vi "Tabelle in die einzelnen Seiten zerlegen.vi"(5 "alternative Datei":string, 6 "Aktion":T1, 7 "Translate.exe":bool, 8 "error in (no error)":errorcluster caption="Fehler (Eingang, kein Fehler)", 9 "Sprachseite":string[][](array[string]), 10 "Eingang":string[][](array[string]), 11 "Index (Seite)":i32) -> (0 "error out":errorcluster caption="Fehler (Ausgang)", 2 "all rows":string[][][](array[string]), 3 "Sprachliste":string[][](array[string]))   [LabVIEW 2020, in "Sprachverwaltung.lvlib"]
doc: "Mit diesen VI kann man die Sprachdatei in den Einzelnen Seiten zerlegen, dabei muss man nur den Index der Seite angeben.\ns"
uses:
  Sprachverwaltung.lvlib
  FGV Aktion Tabelle zerlegen.ctl
  Seiten.ctl
  <vilib>/Utility/file.llb/Read Delimited Spreadsheet (string).vi
  <vilib>/Utility/file.llb/Write Delimited Spreadsheet (string).vi
  Allgemein/allgemeine Sub-VIs.lvlib
  <vilib>/Utility/Data Type/NI_Data Type.lvlib
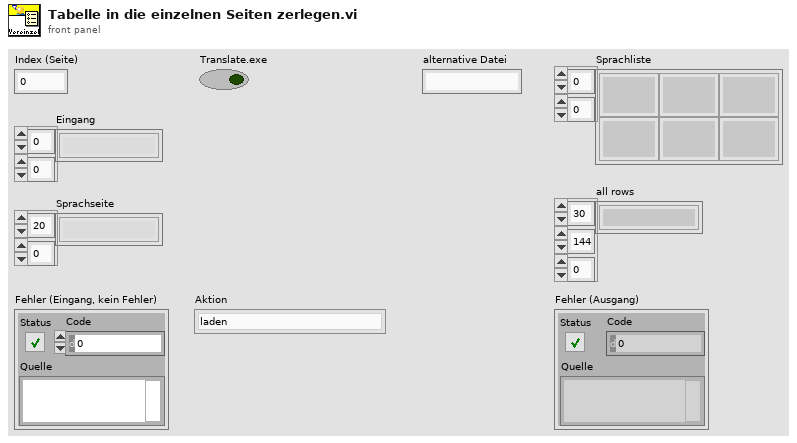
[diagram p1: front panel]
types:
  T1 = typedef "Sprachverwaltung.lvlib/FGV Aktion Tabelle zerlegen.ctl" = enum16{"laden", "vereinzeln", "speichern"}
  T2 = typedef "Sprachverwaltung.lvlib/Seiten.ctl" = enum16{"[ANLAGENGRENZWERTE]", "[LOG KONFIG]", "[GASZUORDNUNG]", "[ANLAGENÜBERSICHT]", "[GRAFIK]", "[CONFIG DIAGRAMME]", "[KONFIGURATION FTIR]", "[GASLISTE VERGLEICHEN]", "[ALGEBRAIC KONFIG]", "[FTIR DIAGNOSE]", "[ERWEITERTE KONFIG]", "[KONFIG AK]", "[STATUS STEUERUNG]", "[PID PARAMETER DRUCK-REGLER]", "[DICHTHEITSTEST]", "[T90 KONFIG]", "[T90]", "[HINTERGRUND]", "[SYSTEM EINSTELLUNGEN V2]", "[COPYRIGHT]", "[STATUSÜBERSICHT]", "[PASSWORTVERWALTUNG]", "[PASSWORT AENDERN]", "[FUNKTIONSTASTEN]", "[PNS]", "[DIAG PNS]", "[RUNTIME MENUE]", "[FAS06]", "[PERMANENT BEREICH]", "[RUNTIME BEENDEN]", "[SPEICHERN]", "[STOERMELDUNGEN]", "[STOERMELDEPUFFER]", "[STOERMELDE-KONFIG]", "[STOERMELDUNGSDATEI]", "[ERWEITERTE GASLISTE]", "[LINEARISIERUNG FTIR]", "[ARN TEST]", "[ARN PROTOKOLL]", "[FEHLER STEUERUNG]", "[POLYNOMKOEFFIZIENTEN]", "[KONFIG LINEARITY VERIFICATION]", "[AUTO LIN VERIFICATION]", "[GRAPHIK KURVEN]", "[EPA DICHTHEITSTEST]", "[REZEPT LADEN]", "[REZEPTWECHSEL]", "[DIAG ZYKLUSZEIT]", "[EPA KONTROLLE PARAMETER]", "[KONFIG GASTEILER]", "[KALIBRIERDATEN LADEN]", "[KONTROLLE PARAMETER VOR LIN]", "[KONFIGURATION KALIBRIERGASE]", "[INTERFERENCE VERIFICATION]", "[INTERFERENCE VERIFICATION 375]", "[INTERFERENCE PROTOKOLL 375]", "[INTERFERENCE PROTOKOLL]", "[INTERFERENCE HILFE]", "[SPUELEN]", "[GASTEILER SPUELEN]", "[GASTEILER KALIBRIEREN]", "[SENSOR KONFIGURATION]", "[KONFIGURATION PMA]", "[KALIBRIERDATEN]", "[KONFIGURATION FID]", "[ABB MANUELL KALIBRIEREN]", "[PMA MANUELL KALIBRIEREN]", "[SPRACHAUSWAHL]", "[SYS LOG HISTORY]", "[SYS LOG STATUS]", "[PNS UEBERSICHT]\t", "[CG TEST]", "[KONFIG CG CHECK]", "[HOVA MAIN]", "[HORIBA GDC]", "[BACKUP]", "[SPAN FAKTOREN]", "[CG POPUP]", "[AUTO CALIBRATION]", "[LIN V2]", "[O2 LEAKTEST]", "[CG TEST RESULT]", "[GASTEILER ABWEICHUNG]", "[EPA LIN CHECK PROTOKOLL]", "[LIN CHECK PROTOKOLL]", "[LEAK CHECK PROTOKOLL]", "[O2 LEAK PROTOKOLL]", "[HANG UP PROTOKOLL]", "[T90 PROTOKOLL]", "[SPRACHEDITOR]", "[SYSLOG CRIO MESSAGES]", "[SYSLOG PC MESSAGES]", "[SYSLOG PROPERTIES MESSAGES]", "[T90 EPA]", "[T90 EPA PDF]", "[SCHEDULER]", "[HINTERGRUND V2]", "[CG TEST PDF]", "[CHILLER EPA TEST]", "[CHILLER EPA PROTOKOLL]", "[FID O2 EPA TEST]", "[FID O2 EPA PROTOKOLL]", "[DRIFT EPA TEST]", "[DRIFT EPA PROTOKOLL]", "[PRE EPA TEST]", "[PRE EPA PROTOKOLL]", "[FID OPTIMIZATION]", "[FID OPTIMIZATION PDF]", "[FID RESPONSE FAKTOR]"}
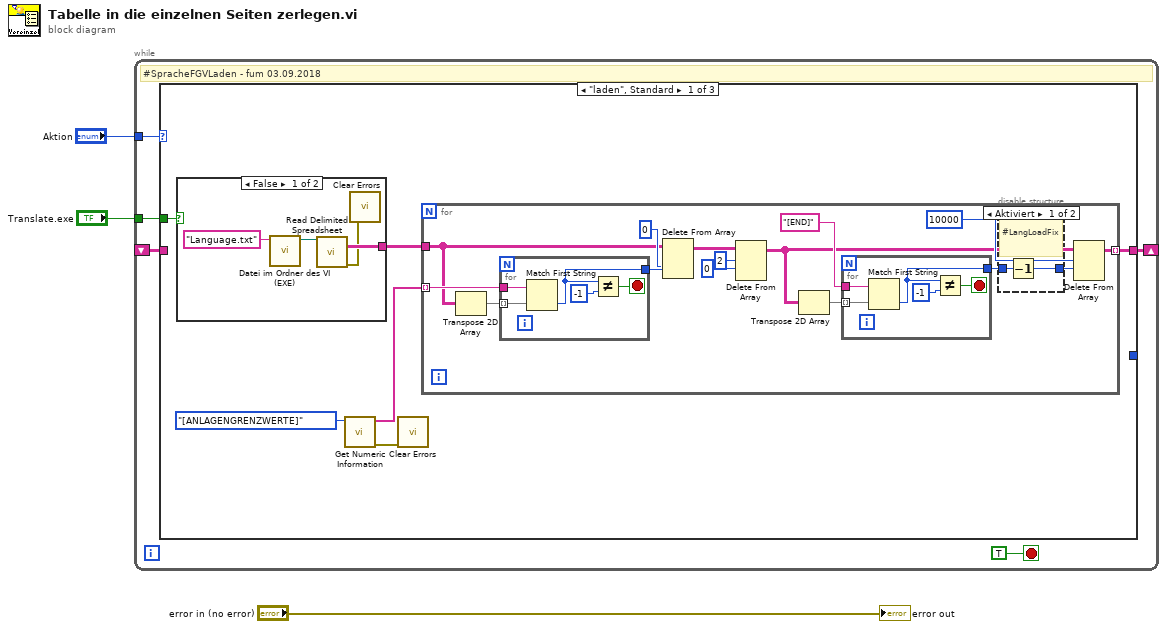
[diagram p0: block diagram]
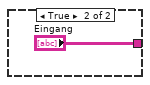
[diagram p3: hidden frame]
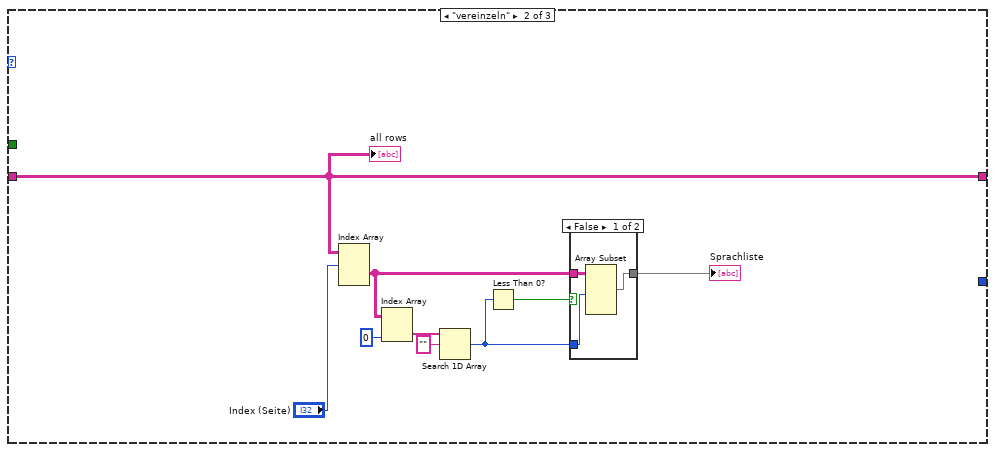
[diagram p4: hidden frame]
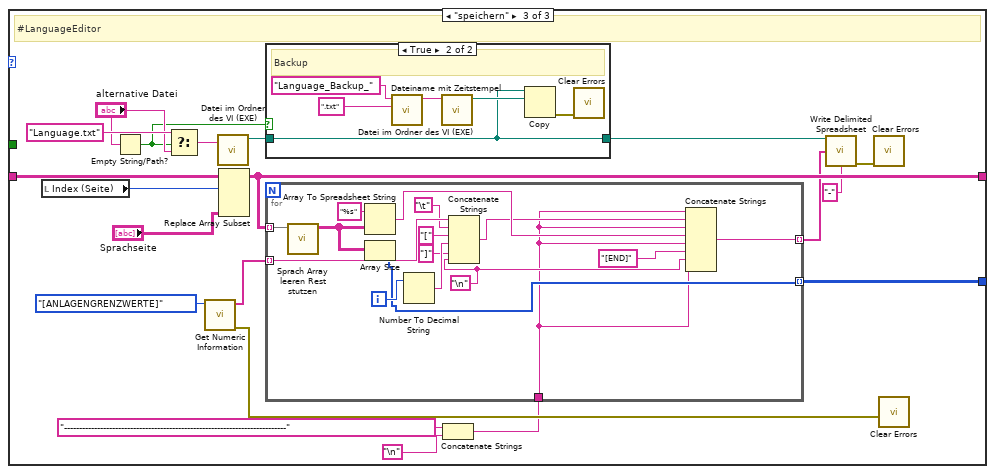
[diagram p6: hidden frame]
diagram:
  n1 = while {
    tunnel: "Aktion" -> [w7]
    tunnel: "Translate.exe" -> [w6]
    shift-right: [w5] -> _
    shift-left: _ -> [w4]
    stop <- TRUE stop-if-true
    # "#SpracheFGVLaden - fum 03.09.2018"
    n2 = case shown="\"laden\", Standard" w7 {
      tunnel: w6 -> [w12 _ _]
      tunnel: [w9 w47 w69] -> w5
      tunnel: w4 -> [_ w47 w76]
      tunnel: [_ _ w65] -> _
      frame "laden", Default {
        n3 = case shown="False" w12 {
          tunnel: [w43 "Eingang"] -> w11
          frame False {
            n4 = call "Datei im Ordner des VI (EXE).vi"("Dateiname"="Language.txt") -> ("Dateipfad im Ordner des Haupt-VIs"=w44:path)  [unwired: 8 in, 2 out]
            n5 = call-poly <vilib>:"Read Delimited Spreadsheet.vi"("file path (dialog if empty)"=w44) -> ("all rows"=w43:string[][], "error out"=w42:errorcluster)  [unwired: 9 in, 4 out]
            n6 = call <vilib>:"Clear Errors.vi"("error in (no error)"=w42) -> ()  [unwired: 5 in, 2 out]
          }
          frame True {
          }
        }
        n7 = call <vilib>:"Get Numeric Information.vi"("variant"=Seiten."[ANLAGENGRENZWERTE]" ("Seiten")) -> ("error out"=w13:errorcluster, "enum names"=w10:string[])  [unwired: 7 in, 2 out]
        n8 = call <vilib>:"Clear Errors.vi"("error in (no error)"=w13) -> ()  [unwired: 5 in, 2 out]
        n9 = for {
          tunnel: w10 -> [w28] mode=indexing
          tunnel: [w22] -> w9 mode=indexing
          tunnel: w11 -> [w17]
          n10 = Transpose 2D Array(2D array=w17) -> (transposed array=w29:string[][])
          n11 = for {
            tunnel: w29 -> [w41] mode=indexing
            tunnel: w28 -> [w40]
            tunnel: [w37] -> w27
            stop <- w38 stop-if-true
            n12 = Match First String(2:w41, 3:w40) -> (0:w37:i32)  [unwired: 1 out]
            n13 = Not Equal?(x=w37, y=-1) -> (x != y?=w38:bool)
          }
          n14 = Delete From Array(array=w17, length=w27, index (row)=0 ("Index (Zeile)")) -> (array with subset deleted=w24:string[][])  [unwired: 1 in, 1 out]
          n15 = Delete From Array(array=w24, length=2 ("Länge"), index (row)=0 ("Index (Zeile)")) -> (array with subset deleted=w20:string[][])  [unwired: 1 in, 1 out]
          n16 = Transpose 2D Array(2D array=w20) -> (transposed array=w25:string[][])
          n17 = for {
            tunnel: w25 -> [w36] mode=indexing
            tunnel: "[END]" ("Regulärer Ausdruck") -> [w35]
            tunnel: [w32] -> w16
            stop <- w33 stop-if-true
            n18 = Match First String(2:w36, 3:w35) -> (0:w32:i32)  [unwired: 1 out]
            n19 = Not Equal?(x=w32, y=-1) -> (x != y?=w33:bool)
          }
          n20 = disable-structure shown="Aktiviert" {
            disable-tunnel: w16 -> [w31 _]
            disable-tunnel: [w30 _] -> w15
            frame Enabled {
              # "#LangLoadFix"
              n21 = Decrement(x=w31) -> (x-1=w30:i32)
            }
            frame Disabled {
            }
          }
          n22 = Delete From Array(array=w20, length=10000 ("Länge"), index (row)=w15) -> (array with subset deleted=w22:string[][])  [unwired: 1 in, 1 out]
        }
      }
      frame "vereinzeln" {
        n23 = Index Array(array=w47, index (dim 0)="Index (Seite)") -> (element=w50:string[][])  [unwired: 2 in]
        n24 = Index Array(array=w50, index (col)=0 ("Deaktivierter Index (Spalte)")) -> (element=w53:string[])  [unwired: 1 in]
        n25 = Search 1D Array(1D array=w53, element="" ("Element")) -> (index of element=w48:i32)  [unwired: 1 in]
        n26 = Less Than 0?(x=w48) -> (x < 0?=w49:bool)
        n27 = case shown="False" w49 {
          tunnel: w50 -> [w58 w59]
          tunnel: [w57 w59] -> w54
          tunnel: w48 -> [w56 _]
          frame False {
            n28 = Array Subset(array=w58, length (row)=w56) -> (w57:string[][])  [unwired: 3 in]
          }
          frame True {
          }
        }
        "Sprachliste" <- w54
        "all rows" <- w47
      }
      frame "speichern" {
        # "#LanguageEditor"
        n29 = local read "Index (Seite)"() -> (w75:i32)
        n30 = Empty String/Path?(string/path="alternative Datei") -> (empty?=w62:bool)
        n31 = Select(t="Language.txt" ("Dateiname"), s=w62, f="alternative Datei") -> (s? t:f=w77:string)
        n32 = call <vilib>:"Get Numeric Information.vi"("variant"=Seiten."[ANLAGENGRENZWERTE]" ("Seiten")) -> ("error out"=w71:errorcluster, "enum names"=w70:string[])  [unwired: 7 in, 2 out]
        n33 = call "Datei im Ordner des VI (EXE).vi"("Dateiname"=w77) -> ("Dateipfad im Ordner des Haupt-VIs"=w61:path)  [unwired: 8 in, 2 out]
        n34 = Replace Array Subset(array=w76, new element="Sprachseite", index (dim 0)=w75) -> (w69:string[][][])  [unwired: 2 in]
        n35 = case shown="True" w62 {
          tunnel: w61 -> [w80 w81]
          tunnel: [w80 w81] -> w60
          frame False {
          }
          frame True {
            # "Backup"
            n36 = call "Dateiname mit Zeitstempel.vi"("Extension in"=".txt" ("alternative Datei"), "File Name in"="Language_Backup_" ("alternative Datei")) -> ("File Name"=w84:string)  [unwired: 9 in]
            n37 = call "Datei im Ordner des VI (EXE).vi"("Dateiname"=w84) -> ("Dateipfad im Ordner des Haupt-VIs"=w83:path)  [unwired: 8 in, 2 out]
            n38 = Copy(10:w83, 11:w81) -> (0:w82:errorcluster)  [unwired: 3 in, 2 out]
            n39 = call <vilib>:"Clear Errors.vi"("error in (no error)"=w82) -> ()  [unwired: 5 in, 2 out]
          }
        }
        n40 = Concatenate Strings("--------------------------------------------------------------------------", "\n") -> (w67:string)
        n41 = for {
          tunnel: w70 -> [w102] mode=indexing
          tunnel: w69 -> [w93] mode=indexing
          tunnel: w67 -> [w88]
          tunnel: [w94] -> w65 mode=indexing
          tunnel: [w87] -> w64 mode=indexing
          i -> [w100]
          w91 = "\n"
          n42 = call "Sprach Array leeren Rest stutzen.vi"("Array in"=w93) -> ("Array out"=w92:string[][])  [unwired: 9 in, 1 out]
          n43 = Array To Spreadsheet String(array=w92, 3:"%s" ("Format-String")) -> (spreadsheet string=w90:string)  [unwired: 1 in]
          n44 = Array Size(array=w92) -> (size(s)=w94:i32[])
          n45 = Number To Decimal String(number=w100) -> (decimal integer string=w98:string)  [unwired: 1 in]
          n46 = Concatenate Strings(w102, "\t", "[", w98, "]", w91) -> (w89:string)
          n47 = Concatenate Strings(w88, w89, w88, w90, w88, "[END]" ("Regulärer Ausdruck"), w91, w88) -> (w87:string)
        }
        n48 = call-poly <vilib>:"Write Delimited Spreadsheet.vi"("file path (dialog if empty)"=w60, "1D data"=w64, "delimiter (\\t)"="-" ("delimiter (\\t)")) -> ("error out"=w73:errorcluster)  [unwired: 11 in, 1 out]
        n49 = call <vilib>:"Clear Errors.vi"("error in (no error)"=w73) -> ()  [unwired: 5 in, 2 out]
        n50 = call <vilib>:"Clear Errors.vi"("error in (no error)"=w71) -> ()  [unwired: 5 in, 2 out]
      }
    }
  }
  "error out" <- "error in (no error)"
